vi "Launch Async Job.vi"(6 "timeout (500 ms)":i32=500, 8 "error in (no error)":errorcluster, 10 "stdin":string, 11 "Job in":refnum<class "Job.lvclass">) -> (0 "error out":errorcluster, 1 "exception":i32, 2 "Job GUID":string, 3 "Job out":refnum<class "Job.lvclass">)   [LabVIEW 2013, in "openCronJob.lvlib" / "Job.lvclass"]
uses:
  Job.lvclass
  Job Details -- cluster.ctl
  Job.lvclass/Job.ctl
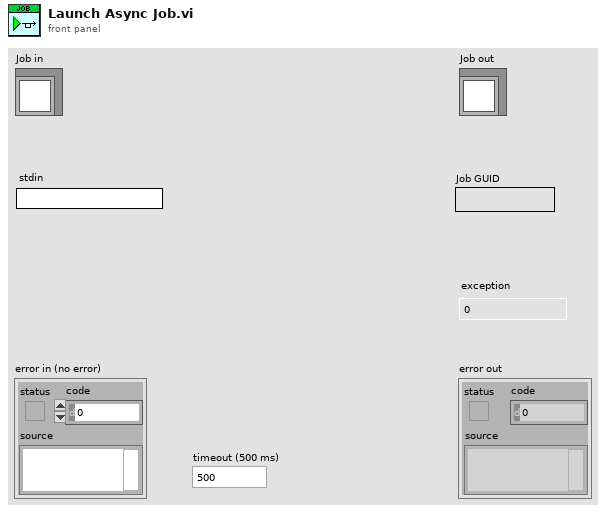
[diagram p1: front panel]
types:
  T1 = typedef "openCronJob.lvlib/Job.lvclass/Job Details -- cluster.ctl" = cluster{"Name":string, "GUID":string, "Abort":refnum<notifier>}
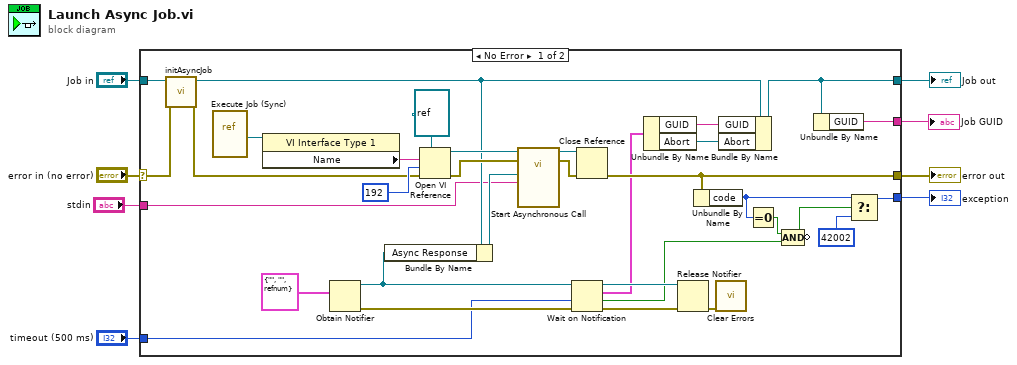
[diagram p0: block diagram]
diagram:
  n1 = case shown="No Error" "error in (no error)" {
    selector: "error in (no error)" -> [w12 w43]
    tunnel: [w28 w43] -> w5
    tunnel: [w16 w42] -> w6
    tunnel: "Job in" -> [w13 w42]
    tunnel: [w26 _] -> w4
    tunnel: "timeout (500 ms)" -> [w21 _]
    tunnel: [w15 _] -> w2
    tunnel: "stdin" -> [w10 _]
    frame No Error {
      n2 = call "initAsyncJob.vi"("error in (no error)"=w12, "Job in"=w13) -> ("error out"=w11:errorcluster, "Job out"=w14:refnum<class "Job.lvclass">)  [unwired: 8 in]
      n3 = vi-ref "Execute Job (Sync).vi"() -> (w41:refnum<vi>)
      n4 = property class="VI Interface Type 1"(reference=w41) -> ("Name"=w40:string)  [unwired: 1 in, 2 out]
      n5 = Obtain Notifier(notification data type=T1 {"Name"="", "GUID"="", "Abort"=refnum} ("Job Details")) -> (notifier out=w34:refnum<notifier>, error out=w32:errorcluster)  [unwired: 3 in, 1 out]
      n6 = Bundle By Name(cluster=w14, "Async Response"=w34) -> (w33:refnum<class "Job.lvclass">)
      n7 = Open VI Reference(type specifier VI Refnum (for type only)=refnum<vi> refnum, vi path=w40, options=192, error in (no error)=w11) -> (vi reference=w38:refnum<vi>, error out=w37:errorcluster)  [unwired: 2 in]
      n8 = call-by-ref "Start Asynchronous Call"(reference=w38, error in=w37, "stdin"=w10, "Job in"=w33) -> (reference out=w36:refnum<vi>, error out=w35:errorcluster)  [unwired: 6 in, 4 out]
      n9 = Wait on Notification(notifier=w34, timeout in ms (-1)=w21, error in (no error)=w32) -> (notifier out=w31:refnum<notifier>, notification=w19:T1, timed out?=w24:bool, error out=w30:errorcluster)  [unwired: 1 in]
      n10 = Close Reference(reference=w36, error in (no error)=w35) -> (error out=w28:errorcluster)
      n11 = Unbundle By Name(w19) -> ("GUID"=w18:string, "Abort"=w17:refnum<notifier>)
      n12 = Release Notifier(notifier=w31, error in (no error)=w30) -> (error out=w29:errorcluster)  [unwired: 1 in, 2 out]
      n13 = Unbundle By Name(w28) -> ("code"=w27:i32)
      n14 = call <vilib>:"Clear Errors.vi"("error in (no error)"=w29) -> ()  [unwired: 6 in, 1 out]
      n15 = Bundle By Name(cluster=w14, "GUID"=w18, "Abort"=w17) -> (w16:refnum<class "Job.lvclass">)
      n16 = Equal To 0?(x=w27) -> (x = 0?=w25:bool)
      n17 = Compound Arithmetic op=AND(w25, w24) -> (invert w23:bool)
      n18 = Unbundle By Name(w16) -> ("GUID"=w15:string)
      n19 = Select(t=w27, s=w23, f=42002 ("timeout in ms (-1)")) -> (s? t:f=w26:i32)
    }
    frame Error {
    }
  }
  "error out" <- w5
  "Job out" <- w6
  "exception" <- w4
  "Job GUID" <- w2
